vi "ClearErr.vi"(8 "error in (no error)":errorcluster caption="错误输入（无错误）", 11 "运行位置":string) -> (0 "error out":errorcluster caption="错误输出")   [LabVIEW 2017]
uses:
  Global System.vi
  <vilib>/Utility/file.llb/Write Delimited Spreadsheet (string).vi
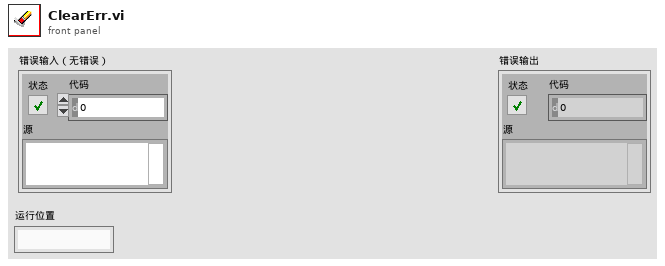
[diagram p1: front panel]
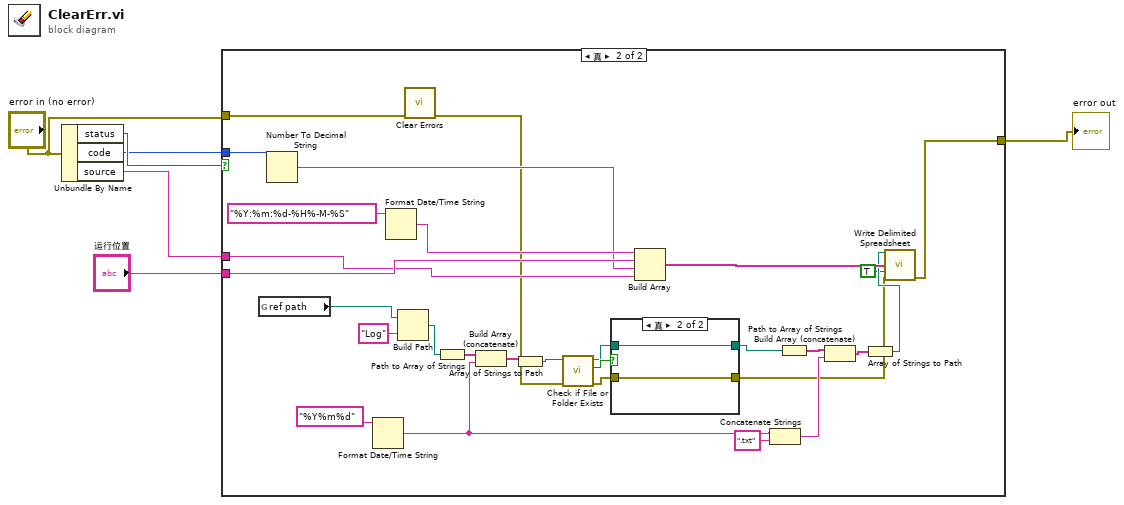
[diagram p0: block diagram]
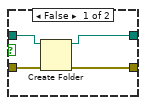
[diagram p3: hidden frame]
diagram:
  n1 = Unbundle By Name("error in (no error)") -> ("status"=w6:bool, "code"=w3:i32, "source"=w1:string)
  n2 = case shown="真" w6 {
    tunnel: "error in (no error)" -> [w7 w12]
    tunnel: [w7 w9] -> w4
    tunnel: w3 -> [_ w34]
    tunnel: "运行位置" -> [_ w32]
    tunnel: w1 -> [_ w30]
    frame False {
    }
    frame True {
      n3 = global read "Global System.vi" "ref path"() -> (w28:path)
      n4 = Number To Decimal String(number=w34) -> (decimal integer string=w31:string)  [unwired: 1 in]
      n5 = Format Date/Time String(time format string (%c)="%Y%m%d" ("时间格式字符串(%c)")) -> (date/time string=w19:string)  [unwired: 2 in]
      n6 = Format Date/Time String(time format string (%c)="%Y:%m:%d-%H%-M-%S" ("时间格式字符串(%c)")) -> (date/time string=w33:string)  [unwired: 2 in]
      n7 = Build Path(base path=w28, name or relative path="Log" ("名称或相对路径")) -> (appended path=w26:path)
      n8 = call <vilib>:"Clear Errors.vi"("error in (no error)"=w12) -> ("error out"=w8:errorcluster)  [unwired: 5 in, 1 out]
      n9 = Path to Array of Strings(0:w26) -> (2:w25:string[])  [unwired: 1 out]
      n10 = Build Array (concatenate)(w25, w19) -> (w24:string[])
      n11 = Array of Strings to Path(0:w24) -> (2:w23:path)  [unwired: 1 in]
      n12 = call <vilib>:"Check if File or Folder Exists.vi"("error in (no error)"=w8, "path"=w23) -> ("error out"=w11:errorcluster, "file or folder exists?"=w22:bool, "dup path"=w21:path)  [unwired: 7 in]
      n13 = case shown="真" w22 {
        tunnel: w21 -> [w40 w42]
        tunnel: [w39 w42] -> w20
        tunnel: w11 -> [w38 w41]
        tunnel: [w37 w41] -> w10
        frame False {
          n14 = Create Folder(path (use dialog)=w40, error in=w38) -> (created path=w39:path, error out=w37:errorcluster)  [unwired: 1 in, 1 out]
        }
        frame True {
        }
      }
      n15 = Build Array(w33, w32, w31, w30) -> (w29:string[])
      n16 = Concatenate Strings(w19, ".txt" ("字符串")) -> (w16:string)
      n17 = Path to Array of Strings(0:w20) -> (2:w17:string[])  [unwired: 1 out]
      n18 = Build Array (concatenate)(w17, w16) -> (w15:string[])
      n19 = Array of Strings to Path(0:w15) -> (2:w14:path)  [unwired: 1 in]
      n20 = call-poly <vilib>:"Write Delimited Spreadsheet.vi"("file path (dialog if empty)"=w14, "1D data"=w29, "append to file? (new file:F)"=TRUE, "error in (no error)"=w10) -> ("error out"=w9:errorcluster)  [unwired: 10 in, 1 out]
    }
  }
  "error out" <- w4
